vi "CANOpen_Main_Scale TPDO Data.vi"(8 "error in (no error)":errorcluster, 9 "PDO Settings":T1={"Parameters"=[], "PDO Channel"=1, "Start Index"=0, "Length"=0} {"PDO Channel" items=["PDO 1", "PDO 2", "PDO 3", "PDO 4"]; "Parameters"."Bit Offset" max=8 step=1; "Parameters"."Byte Offset" max=8 step=1}, 10 "timestamp":timestamp, 11 "data":u8[](array[numeric])) -> (0 "error out":errorcluster, 2 "Array":dbl[](array[numeric]), 3 "Timestamp":timestamp=timestamp(11705972400 s since 1904-01-01))   [LabVIEW 2021, in "CANOpen Addon Engine.lvlib"]
uses:
  Shared/CANOpen_PDO Settings.ctl
  Shared/CANOpen_PDO Parameter Settings.ctl
  Shared/CANOpen_PDO Data Type.ctl
  System Explorer/SubVIs/CANopen Byte Order.ctl
  <vilib>/CANopenLib/CANOPEN.llb/CANopen Fetch from Data [U8].vi
  <vilib>/CANopenLib/CANOPEN.llb/CANopen Fetch from Data [U16].vi
  <vilib>/CANopenLib/CANOPEN.llb/CANopen Fetch from Data [U32].vi
  <vilib>/CANopenLib/CANOPEN.llb/CANopen Fetch from Data [I16].vi
  <vilib>/CANopenLib/CANOPEN.llb/CANopen Fetch from Data [I32].vi
  <vilib>/CANopenLib/CANOPEN.llb/CANopen Fetch from Data [SGL].vi
  <vilib>/CANopenLib/CANOPEN.llb/CANopen Fetch from Data [DBL].vi
  <vilib>/CANopenLib/CANOPEN.llb/CANopen Fetch from Data [I8].vi
  CANOpen Addon Engine.lvlib
  Shared/CANOpen Addon Shared.lvlib
  System Explorer/CANOpen Addon System Explorer.lvlib
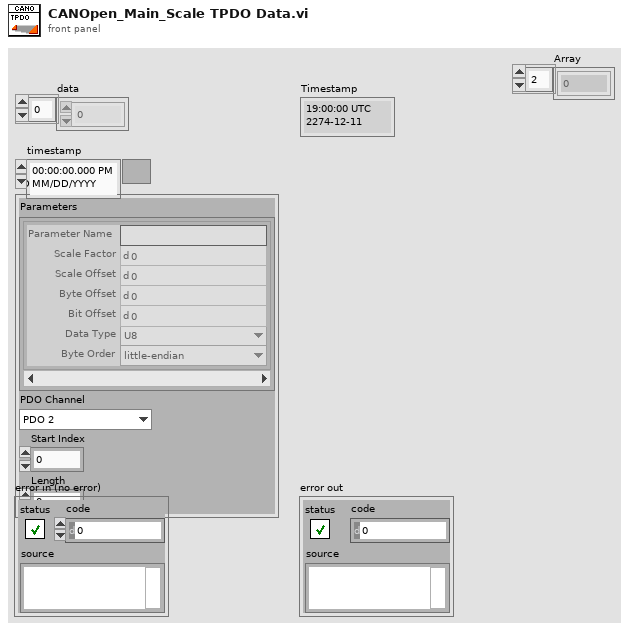
[diagram p1: front panel]
types:
  T1 = typedef "CANOpen Addon Shared.lvlib/CANOpen_PDO Settings.ctl" = cluster{"Parameters":T2[], "PDO Channel":u8, "Start Index":u32, "Length":u32}
  T2 = typedef "CANOpen Addon Shared.lvlib/CANOpen_PDO Parameter Settings.ctl" = cluster{"Parameter Name":string, "Scale Factor":dbl, "Scale Offset":dbl, "Byte Offset":u8, "Bit Offset":u8, "Data Type":T3, "Byte Order":T4}
  T3 = typedef "CANOpen Addon Shared.lvlib/CANOpen_PDO Data Type.ctl" = enum16{"U8", "U16", "U32", "I8", "I16", "I32", "Single", "Double", "Boolean"}
  T4 = typedef "CANOpen Addon System Explorer.lvlib/CANopen Byte Order.ctl" = enum16{"big-endian network order", "little-endian"}
  T5 = enum16{"big-endian, network order", "native, host order", "little-endian"}
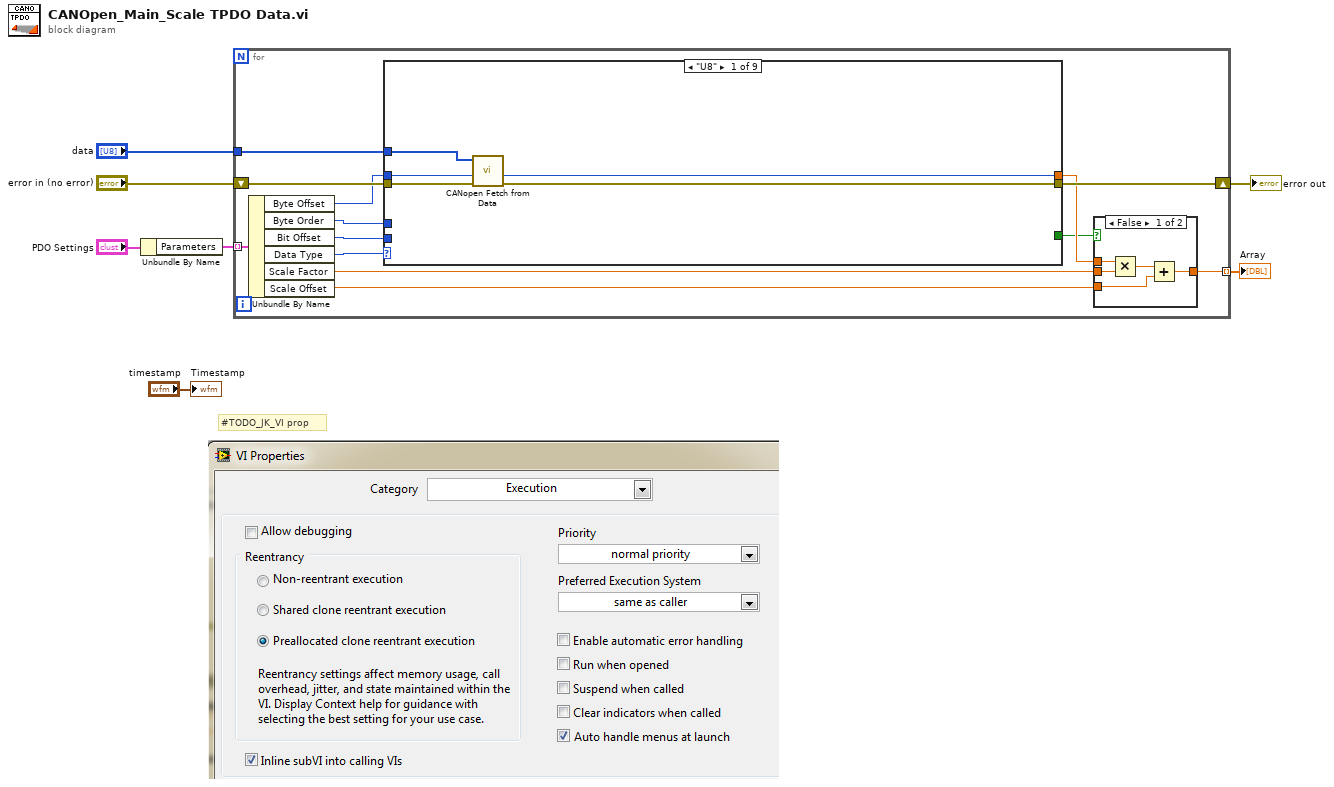
[diagram p0: block diagram]
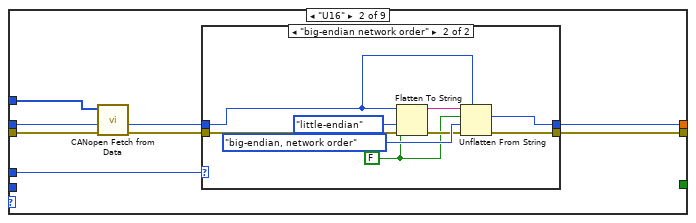
[diagram p3: hidden frame]
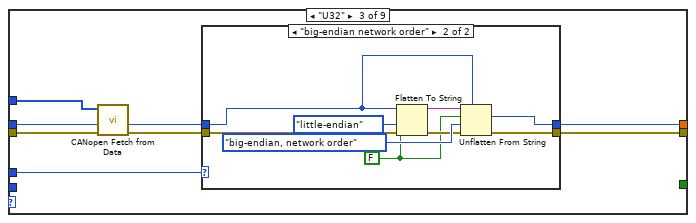
[diagram p5: hidden frame]
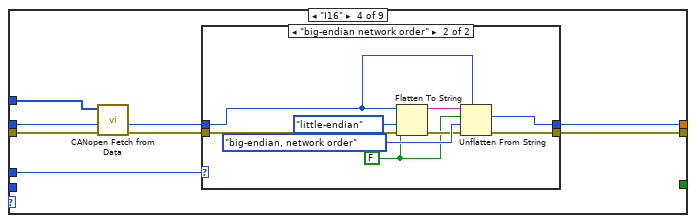
[diagram p7: hidden frame]
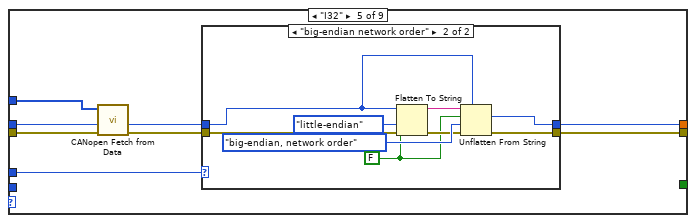
[diagram p9: hidden frame]
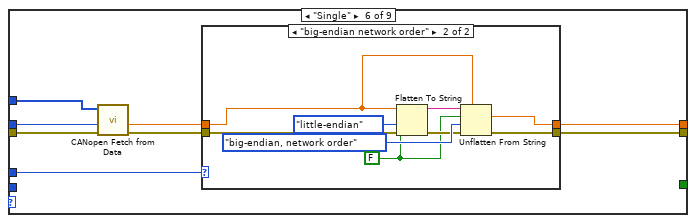
[diagram p11: hidden frame]
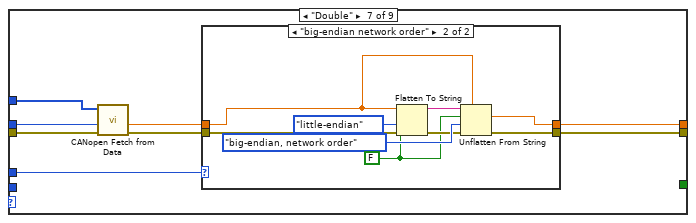
[diagram p13: hidden frame]
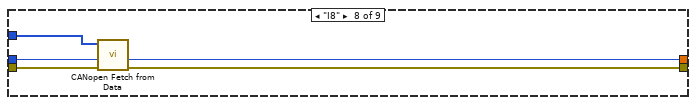
[diagram p15: hidden frame]
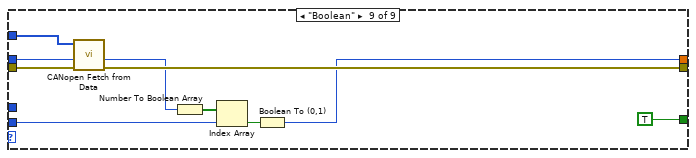
[diagram p16: hidden frame]
diagram:
  # "#TODO_JK_VI prop"
  n1 = Unbundle By Name("PDO Settings") -> ("Parameters"=w2:T2[])
  n2 = for {
    tunnel: "data" -> [w19]
    tunnel: w2 -> [w17] mode=indexing
    shift-right: [w18] -> w6
    shift-left: "error in (no error)" -> [w20]
    tunnel: [w10] -> w1 mode=indexing
    n3 = Unbundle By Name(w17) -> ("Byte Offset"=w15:u8, "Byte Order"=w9:T4, "Bit Offset"=w14:u8, "Data Type"=w16:T3, "Scale Factor"=w12:dbl, "Scale Offset"=w11:dbl)
    n4 = case shown="\"U8\"" w16 {
      tunnel: w20 -> [w31 w39 w58 w77 w96 w115 w134 w150 w160]
      tunnel: w19 -> [w30 w38 w57 w76 w95 w114 w133 w149 w159]
      tunnel: [w29 w33 w52 w71 w90 w109 w128 w148 w158] -> w18
      tunnel: w15 -> [w28 w37 w56 w75 w94 w113 w132 w147 w157]
      tunnel: [w27 w35 w54 w73 w92 w111 w130 w146 w152] -> w13
      tunnel: w14 -> [_ _ _ _ _ _ _ _ w155]
      tunnel: w9 -> [_ w32 w51 w70 w89 w108 w127 _ _]
      tunnel: [_ _ _ _ _ _ _ _ TRUE] -> w8
      frame "U8" {
        n5 = call-poly <vilib>:"CANopen Fetch from Data.vi"("error in (no error)"=w31, "offset (0)"=w28, "CANopen data in"=w30) -> ("error out"=w29:errorcluster, "unsigned 8-bit integer"=w27:u8)  [unwired: 6 in, 1 out]
      }
      frame "U16" {
        n6 = call-poly <vilib>:"CANopen Fetch from Data.vi"("error in (no error)"=w39, "offset (0)"=w37, "CANopen data in"=w38) -> ("error out"=w34:errorcluster, "unsigned 16-bit integer"=w36:u16)  [unwired: 6 in, 1 out]
        n7 = case shown="\"big-endian network order\"" w32 {
          tunnel: w36 -> [w40 w46]
          tunnel: [w40 w45] -> w35
          tunnel: w34 -> [w41 w44]
          tunnel: [w41 w43] -> w33
          frame "little-endian", Default {
          }
          frame "big-endian network order" {
            w42 = FALSE ("prepend array or string size? (T)")
            n8 = Flatten To String(anything=w46, prepend array or string size? (T)=w42, byte order (0:big-endian, network order)=T5."little-endian", error in (no error)=w44) -> (data string=w49:string, error out=w47:errorcluster)  [unwired: 1 out]
            n9 = Unflatten From String(type=w46, binary string=w49, data includes array or string size? (T)=w42, byte order (0:big-endian, network order)=T5."big-endian, network order", error in (no error)=w47) -> (value=w45:u16, error out=w43:errorcluster)  [unwired: 1 out]
          }
        }
      }
      frame "U32" {
        n10 = call-poly <vilib>:"CANopen Fetch from Data.vi"("error in (no error)"=w58, "offset (0)"=w56, "CANopen data in"=w57) -> ("error out"=w53:errorcluster, "unsigned 32-bit integer"=w55:u32)  [unwired: 6 in, 1 out]
        n11 = case shown="\"big-endian network order\"" w51 {
          tunnel: w55 -> [w59 w65]
          tunnel: [w59 w64] -> w54
          tunnel: w53 -> [w60 w63]
          tunnel: [w60 w62] -> w52
          frame "little-endian", Default {
          }
          frame "big-endian network order" {
            w61 = FALSE ("prepend array or string size? (T)")
            n12 = Flatten To String(anything=w65, prepend array or string size? (T)=w61, byte order (0:big-endian, network order)=T5."little-endian", error in (no error)=w63) -> (data string=w68:string, error out=w66:errorcluster)  [unwired: 1 out]
            n13 = Unflatten From String(type=w65, binary string=w68, data includes array or string size? (T)=w61, byte order (0:big-endian, network order)=T5."big-endian, network order", error in (no error)=w66) -> (value=w64:u32, error out=w62:errorcluster)  [unwired: 1 out]
          }
        }
      }
      frame "I16" {
        n14 = call-poly <vilib>:"CANopen Fetch from Data.vi"("error in (no error)"=w77, "offset (0)"=w75, "CANopen data in"=w76) -> ("error out"=w72:errorcluster, "signed 16-bit integer"=w74:i16)  [unwired: 6 in, 1 out]
        n15 = case shown="\"big-endian network order\"" w70 {
          tunnel: w74 -> [w78 w84]
          tunnel: [w78 w83] -> w73
          tunnel: w72 -> [w79 w82]
          tunnel: [w79 w81] -> w71
          frame "little-endian", Default {
          }
          frame "big-endian network order" {
            w80 = FALSE ("prepend array or string size? (T)")
            n16 = Flatten To String(anything=w84, prepend array or string size? (T)=w80, byte order (0:big-endian, network order)=T5."little-endian", error in (no error)=w82) -> (data string=w87:string, error out=w85:errorcluster)  [unwired: 1 out]
            n17 = Unflatten From String(type=w84, binary string=w87, data includes array or string size? (T)=w80, byte order (0:big-endian, network order)=T5."big-endian, network order", error in (no error)=w85) -> (value=w83:i16, error out=w81:errorcluster)  [unwired: 1 out]
          }
        }
      }
      frame "I32" {
        n18 = call-poly <vilib>:"CANopen Fetch from Data.vi"("error in (no error)"=w96, "offset (0)"=w94, "CANopen data in"=w95) -> ("error out"=w91:errorcluster, "signed 32-bit integer"=w93:i32)  [unwired: 6 in, 1 out]
        n19 = case shown="\"big-endian network order\"" w89 {
          tunnel: w93 -> [w97 w103]
          tunnel: [w97 w102] -> w92
          tunnel: w91 -> [w98 w101]
          tunnel: [w98 w100] -> w90
          frame "little-endian", Default {
          }
          frame "big-endian network order" {
            w99 = FALSE ("prepend array or string size? (T)")
            n20 = Flatten To String(anything=w103, prepend array or string size? (T)=w99, byte order (0:big-endian, network order)=T5."little-endian", error in (no error)=w101) -> (data string=w106:string, error out=w104:errorcluster)  [unwired: 1 out]
            n21 = Unflatten From String(type=w103, binary string=w106, data includes array or string size? (T)=w99, byte order (0:big-endian, network order)=T5."big-endian, network order", error in (no error)=w104) -> (value=w102:i32, error out=w100:errorcluster)  [unwired: 1 out]
          }
        }
      }
      frame "Single" {
        n22 = call-poly <vilib>:"CANopen Fetch from Data.vi"("error in (no error)"=w115, "offset (0)"=w113, "CANopen data in"=w114) -> ("error out"=w110:errorcluster, "4-byte single"=w112:sgl)  [unwired: 6 in, 1 out]
        n23 = case shown="\"big-endian network order\"" w108 {
          tunnel: w112 -> [w116 w122]
          tunnel: [w116 w121] -> w111
          tunnel: w110 -> [w117 w120]
          tunnel: [w117 w119] -> w109
          frame "little-endian", Default {
          }
          frame "big-endian network order" {
            w118 = FALSE ("prepend array or string size? (T)")
            n24 = Flatten To String(anything=w122, prepend array or string size? (T)=w118, byte order (0:big-endian, network order)=T5."little-endian", error in (no error)=w120) -> (data string=w125:string, error out=w123:errorcluster)  [unwired: 1 out]
            n25 = Unflatten From String(type=w122, binary string=w125, data includes array or string size? (T)=w118, byte order (0:big-endian, network order)=T5."big-endian, network order", error in (no error)=w123) -> (value=w121:sgl, error out=w119:errorcluster)  [unwired: 1 out]
          }
        }
      }
      frame "Double" {
        n26 = call-poly <vilib>:"CANopen Fetch from Data.vi"("error in (no error)"=w134, "offset (0)"=w132, "CANopen data in"=w133) -> ("error out"=w129:errorcluster, "8-byte double"=w131:dbl)  [unwired: 6 in, 1 out]
        n27 = case shown="\"big-endian network order\"" w127 {
          tunnel: w131 -> [w135 w141]
          tunnel: [w135 w140] -> w130
          tunnel: w129 -> [w136 w139]
          tunnel: [w136 w138] -> w128
          frame "little-endian", Default {
          }
          frame "big-endian network order" {
            w137 = FALSE ("prepend array or string size? (T)")
            n28 = Flatten To String(anything=w141, prepend array or string size? (T)=w137, byte order (0:big-endian, network order)=T5."little-endian", error in (no error)=w139) -> (data string=w144:string, error out=w142:errorcluster)  [unwired: 1 out]
            n29 = Unflatten From String(type=w141, binary string=w144, data includes array or string size? (T)=w137, byte order (0:big-endian, network order)=T5."big-endian, network order", error in (no error)=w142) -> (value=w140:dbl, error out=w138:errorcluster)  [unwired: 1 out]
          }
        }
      }
      frame "I8" {
        n30 = call-poly <vilib>:"CANopen Fetch from Data.vi"("error in (no error)"=w150, "offset (0)"=w147, "CANopen data in"=w149) -> ("error out"=w148:errorcluster, "signed 8-bit integer"=w146:i8)  [unwired: 6 in, 1 out]
      }
      frame "Boolean" {
        n31 = call-poly <vilib>:"CANopen Fetch from Data.vi"("error in (no error)"=w160, "offset (0)"=w157, "CANopen data in"=w159) -> ("error out"=w158:errorcluster, "unsigned 8-bit integer"=w153:u8)  [unwired: 6 in, 1 out]
        n32 = Number To Boolean Array(number=w153) -> (Boolean array=w156:bool[])
        n33 = Index Array(array=w156, index=w155) -> (element=w154:bool)
        n34 = Boolean To (0,1)(Boolean=w154) -> (0, 1=w152:i16)
      }
    }
    n35 = case shown="False" w8 {
      tunnel: w13 -> [w25 w26]
      tunnel: w12 -> [w24 _]
      tunnel: w11 -> [w22 _]
      tunnel: [w21 w26] -> w10
      frame False {
        n36 = Multiply(x=w25, y=w24) -> (x*y=w23:dbl)
        n37 = Add(x=w23, y=w22) -> (x+y=w21:dbl)
      }
      frame True {
      }
    }
  }
  "error out" <- w6
  "Array" <- w1
  "Timestamp" <- "timestamp"
